vi "U3 PWM16 and Duty Cycle.vi"(8 "error in":errorcluster, 9 "PWM Duty Cycle [%]":dbl=50.0 format="%.4f") -> (0 "error out":errorcluster)   [LabVIEW 2021]
panel:
  out "Measured Duty Cycle [%]":dbl format="%.8f"
  out "Low Time (s)":dbl format="%.8f"
  out "Low Time (Clocks)":u16
  out "High Time (s)":dbl format="%.8f"
  out "High Time (Clocks)":u16
  out "Timer1 Value Read":u32
  in  "FirstFound":bool=TRUE
  in  "Address":string="1"
  out "Error Message":string
  # "Demonstrates 1 timer channel of 16-bit PWM output with a frequency of 40.6 Hz, and 1 timer channel doing\nduty cycle input.  Short FIO4 (PWM output) to FIO5 (duty cycle input) and then you can measure the duty\ncycle of the output."
  # "This VI passes a timer\nbase clock constant that\nis valid for hardware V1.21+.\nFor hardware V1.20 change\nLJ_tc48MHZ_DIV to LJ_tc24MHZ_DIV."
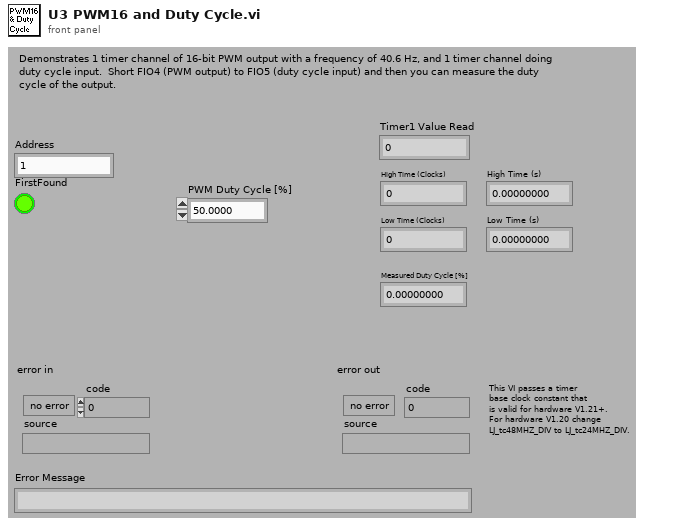
[diagram p1: front panel]
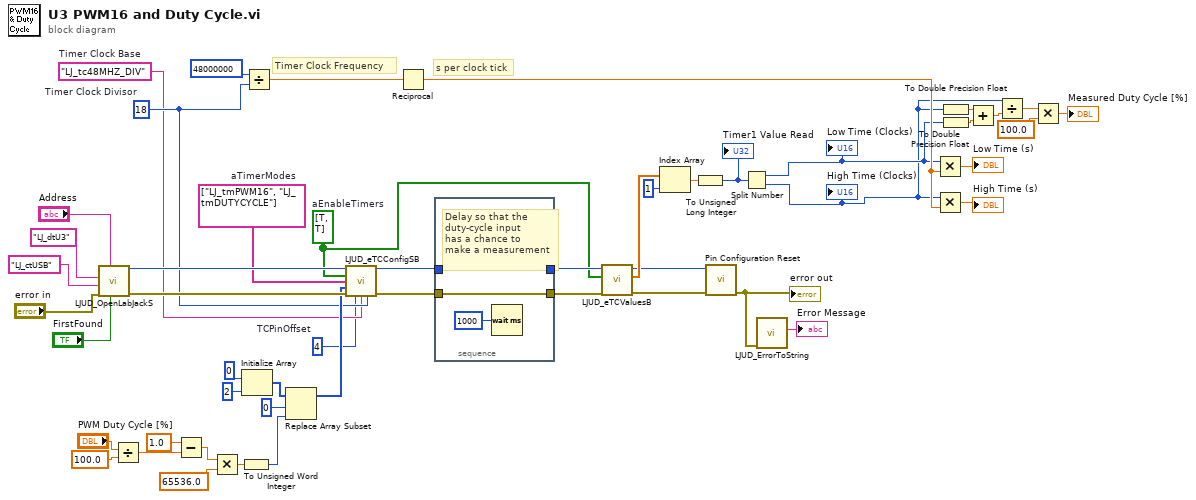
[diagram p0: block diagram]
diagram:
  w2 = 4  # TCPinOffset
  w1 = bool[] [TRUE, TRUE]  # aEnableTimers
  w4 = 18  # Timer Clock Divisor
  w3 = "LJ_tc48MHZ_DIV"  # Timer Clock Base
  w6 = string[] ["LJ_tmPWM16", "LJ_tmDUTYCYCLE"]  # aTimerModes
  # "s per clock tick"
  # "Timer Clock Frequency"
  n1 = call "LJUD_OpenLabJackS.vi"("FirstFound"="FirstFound", "Address"="Address", "error in"="error in", "ConnectionType"="LJ_ctUSB", "DeviceType"="LJ_dtU3") -> ("error out"=w8:errorcluster, "Handle"=w7:i32)  [unwired: 4 in, 1 out]
  n2 = Divide(x="PWM Duty Cycle [%]", y=100.0) -> (x/y=w45:dbl)
  n3 = Subtract(x=1.0, y=w45) -> (x-y=w43:dbl)
  n4 = Multiply(x=w43, y=65536.0) -> (x*y=w33:dbl)
  n5 = To Unsigned Word Integer(number=w33) -> (unsigned 16bit integer=w32:u16)
  n6 = Initialize Array(u16 0 ("PWM Timer Value"), 2 ("Dimension Size")) -> (w37:u16[])
  n7 = Divide(x=48000000, y=w4) -> (x/y=w26:dbl)
  n8 = Replace Array Subset(array=w37, new element=w32, index=0 ("Index")) -> (w5:u16[])
  n9 = call "LJUD_eTCConfigSB.vi"("Handle In"=w7, "aEnableTimers"=w1, "aTimerModes"=w6, "aTimerValues"=w5, "error in"=w8, "TCPinOffset"=w2, "TimerClockBase"=w3, "TimerClockDivisor"=w4) -> ("Handle Out"=w10:i32, "error out"=w9:errorcluster)  [unwired: 6 in]
  n10 = Reciprocal(x=w26) -> (1/x=w25:dbl)
  n11 = stacked-sequence {
    tunnel: w9 -> [w53]
    tunnel: [w53] -> w31
    tunnel: w10 -> [w52]
    tunnel: [w52] -> w30
    frame #0 {
      # "Delay so that the\nduty-cycle input\nhas a chance to\nmake a measurement"
      n12 = Wait (ms)(milliseconds to wait=u32 1000) -> ()  [unwired: 1 out]
    }
  }
  n13 = call "LJUD_eTCValuesB.vi"("error in"=w31, "aReadTimers"=w1, "Handle In"=w30) -> ("error out"=w12:errorcluster, "aTimerValues Read"=w29:dbl[], "Handle Out"=w13:i32)  [unwired: 5 in, 1 out]
  n14 = Index Array(array=w29, index=1 ("Index")) -> (element=w14:dbl)
  n15 = To Unsigned Long Integer(number=w14) -> (unsigned 32bit integer=w27:u32)
  "Timer1 Value Read" <- w27
  n16 = call "Pin Configuration Reset.vi"("error in"=w12, "Handle In"=w13) -> ("error out"=w11:errorcluster)  [unwired: 8 in, 1 out]
  "error out" <- w11
  n17 = Split Number(x=w27) -> (hi(x)=w19:u16, lo(x)=w18:u16)
  "High Time (Clocks)" <- w18
  "Low Time (Clocks)" <- w19
  n18 = call "LJUD_ErrorToString.vi"("error in"=w11) -> ("String"=→"Error Message":string)  [unwired: 10 in]
  n19 = Multiply(x=w19, y=w25) -> (x*y=→"Low Time (s)":dbl)
  n20 = Multiply(x=w18, y=w25) -> (x*y=→"High Time (s)":dbl)
  n21 = To Double Precision Float(number=w18) -> (double precision float=w20:dbl)
  n22 = To Double Precision Float(number=w19) -> (double precision float=w21:dbl)
  n23 = Add(x=w20, y=w21) -> (x+y=w22:dbl)
  n24 = Divide(x=w18, y=w22) -> (x/y=w17:dbl)
  n25 = Multiply(x=w17, y=100.0) -> (x*y=→"Measured Duty Cycle [%]":dbl)
